vi "U8 to U32.vi"(1 "Byte1":u8, 2 "Byte2":u8, 3 "Byte3":u8, 4 "Byte4":u8, 7 "MSB first (T)":bool=TRUE) -> (16 "U32":u32)   [LabVIEW 2013, in "VRI.lvlib"]
uses:
  VRI.lvlib
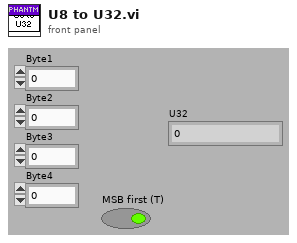
[diagram p1: front panel]
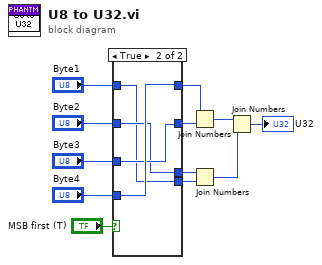
[diagram p0: block diagram]
diagram:
  n1 = case shown="True" "MSB first (T)" {
    tunnel: "Byte1" -> [w13 w17]
    tunnel: "Byte3" -> [w15 w19]
    tunnel: "Byte4" -> [w16 w20]
    tunnel: "Byte2" -> [w14 w18]
    tunnel: [w13 w20] -> w5
    tunnel: [w14 w19] -> w4
    tunnel: [w15 w18] -> w3
    tunnel: [w16 w17] -> w2
    frame False {
    }
    frame True {
    }
  }
  n2 = Join Numbers(hi=w5, lo=w4) -> ((hi.lo)=w10:u16)
  n3 = Join Numbers(hi=w3, lo=w2) -> ((hi.lo)=w11:u16)
  n4 = Join Numbers(hi=w10, lo=w11) -> ((hi.lo)=→"U32":u32)
